vi "Change Enum Strings.vi"(8 "error in (no error)":errorcluster, 10 "Strings []":string[](array[string]), 11 "vi path":path) -> (0 "error out":errorcluster)   [LabVIEW 2021]
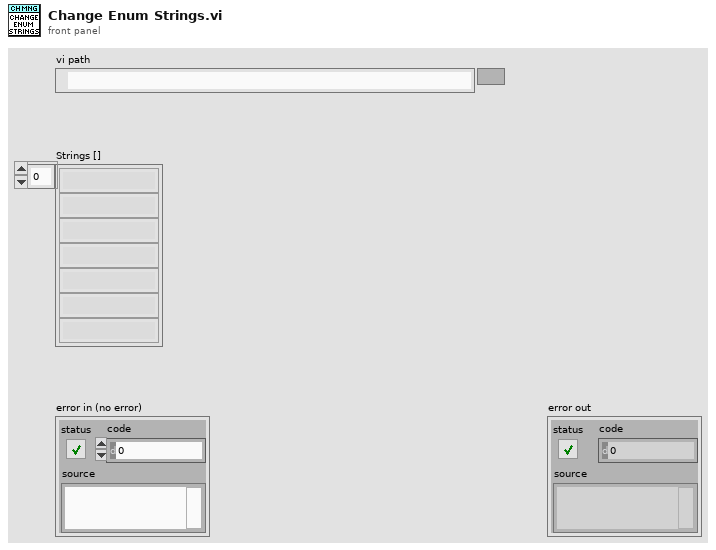
[diagram p1: front panel]
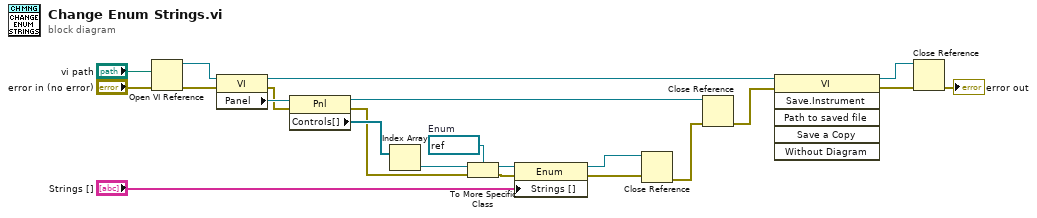
[diagram p0: block diagram]
diagram:
  w17 = refnum<vi> refnum  # Enum
  n1 = Open VI Reference(vi path="vi path", error in (no error)="error in (no error)") -> (vi reference=w22:refnum<vi>, error out=w21:errorcluster)  [unwired: 4 in]
  n2 = property class="VI"(reference=w22, error in=w21) -> (reference out=w8:refnum<vi>, error out=w12:errorcluster, "Panel"=w20:refnum<vi>)
  n3 = property class="Pnl"(reference=w20, error in=w12) -> (reference out=w10:refnum<vi>, error out=w13:errorcluster, "Controls[]"=w19:refnum<vi>[])
  n4 = Index Array(array=w19) -> (element=w18:refnum<vi>)  [unwired: 1 in]
  n5 = To More Specific Class(target class=w17, reference=w18, error in=w13) -> (specific class reference=w16:refnum<vi>, error out=w14:errorcluster)
  n6 = property class="Enum"(reference=w16, error in=w14, "Strings []"="Strings []") -> (reference out=w11:refnum<vi>, error out=w15:errorcluster)
  n7 = Close Reference(reference=w11, error in (no error)=w15) -> (error out=w9:errorcluster)
  n8 = Close Reference(reference=w10, error in (no error)=w9) -> (error out=w7:errorcluster)
  n9 = invoke class="VI" method="Save.Instrument"(reference=w8, error in=w7) -> (reference out=w6:refnum<vi>, error out=w5:errorcluster)  [unwired: 4 in, 4 out]
  n10 = Close Reference(reference=w6, error in (no error)=w5) -> (error out=→"error out":errorcluster)
